vi "roll_indicator_calc.vi"(4 "Roll (in)":i32) -> (1 "Roll Indicator (out)":cluster{"Roll ctrl":i32, i32})   [LabVIEW 8.6]
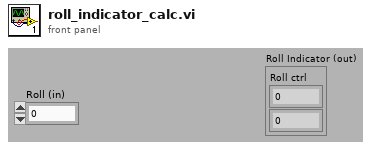
[diagram p1: front panel]
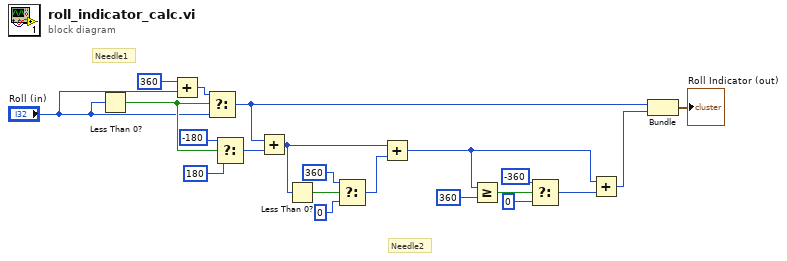
[diagram p0: block diagram]
diagram:
  # "Needle2"
  # "Needle1"
  n1 = Less Than 0?(x="Roll (in)") -> (x < 0?=w5:bool)
  n2 = Add(x=360, y="Roll (in)") -> (x+y=w2:i32)
  n3 = Select(t=w2, s=w5, f="Roll (in)") -> (s? t:f=w9:i32)
  n4 = Select(t=-180 ("y"), s=w5, f=180 ("y")) -> (s? t:f=w8:i32)
  n5 = Add(x=w9, y=w8) -> (x+y=w14:i32)
  n6 = Less Than 0?(x=w14) -> (x < 0?=w10:bool)
  n7 = Select(t=360, s=w10, f=0) -> (s? t:f=w11:i32)
  n8 = Add(x=w14, y=w11) -> (x+y=w20:i32)
  n9 = Greater Or Equal?(x=w20, y=360) -> (x >= y?=w16:bool)
  n10 = Select(t=-360, s=w16, f=0) -> (s? t:f=w19:i32)
  n11 = Add(x=w20, y=w19) -> (x+y=w21:i32)
  n12 = Bundle("Roll (in)"=w9, w21) -> (→"Roll Indicator (out)":cluster{"Roll (in)":i32, i32})  [unwired: 1 in]
